vi "Wheel Pos Auto Adjust.vi"(7 "Action":enum16{"Initialize", "Analyzing", "Choosing"}(ring)=enum."Analyzing", 8 "error in":errorcluster, 10 "Wheel position":string, 11 "Refnum in":T2) -> (0 "error out":errorcluster, 1 "Best wheel position":string, 2 "No position match?":bool, 3 "Refnum out":T2, 4 "Laser position score":T1(array[cluster]))   [LabVIEW 2019, in "Image.lvlib"]
uses:
  Image.lvlib
  <vilib>/vision/Image Controls.llb/IMAQ Image.ctl
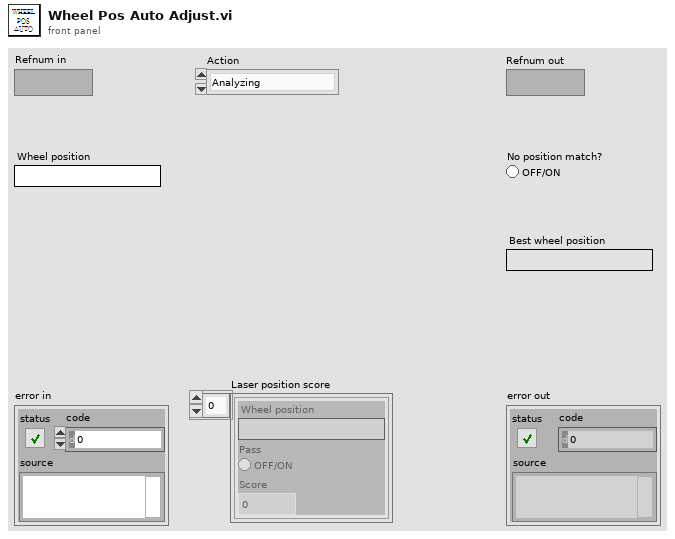
[diagram p1: front panel]
types:
  T1 = cluster{"Wheel position":string, "Pass":bool, "Score":i32}[]
  T2 = typedef "IMAQ Image.ctl" = refnum<image>
  T3 = cluster{"Laser position score":cluster{"Wheel position":string, "Pass":bool, "Score":i32}[], "No position match?":bool, "Best wheel position":string}
  T4 = cluster{"Wheel position":string, "Pass":bool, "Score":i32}
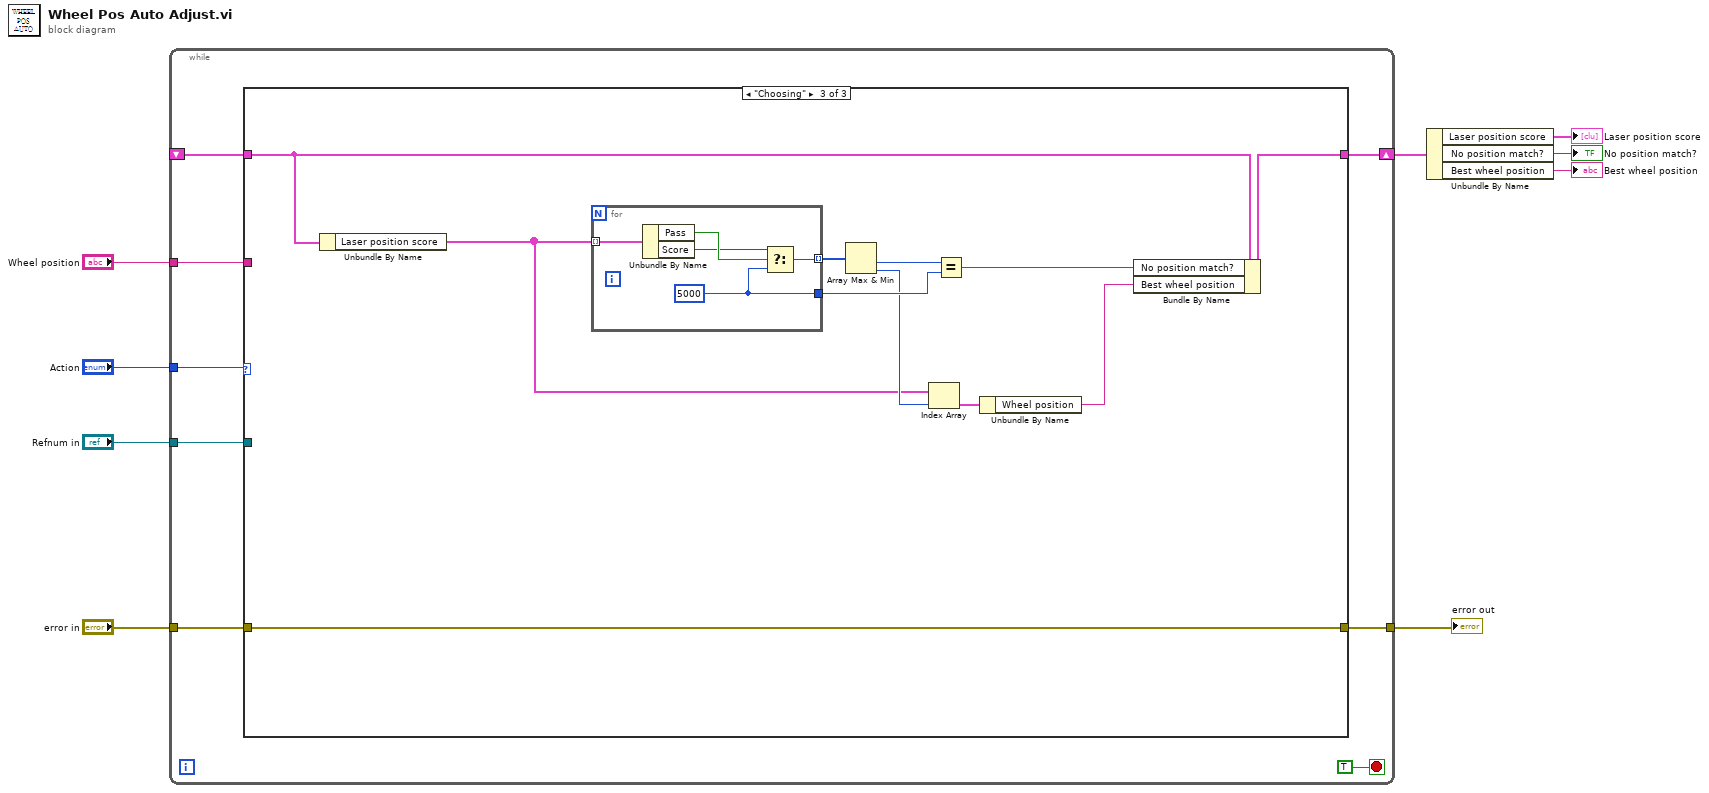
[diagram p0: block diagram]
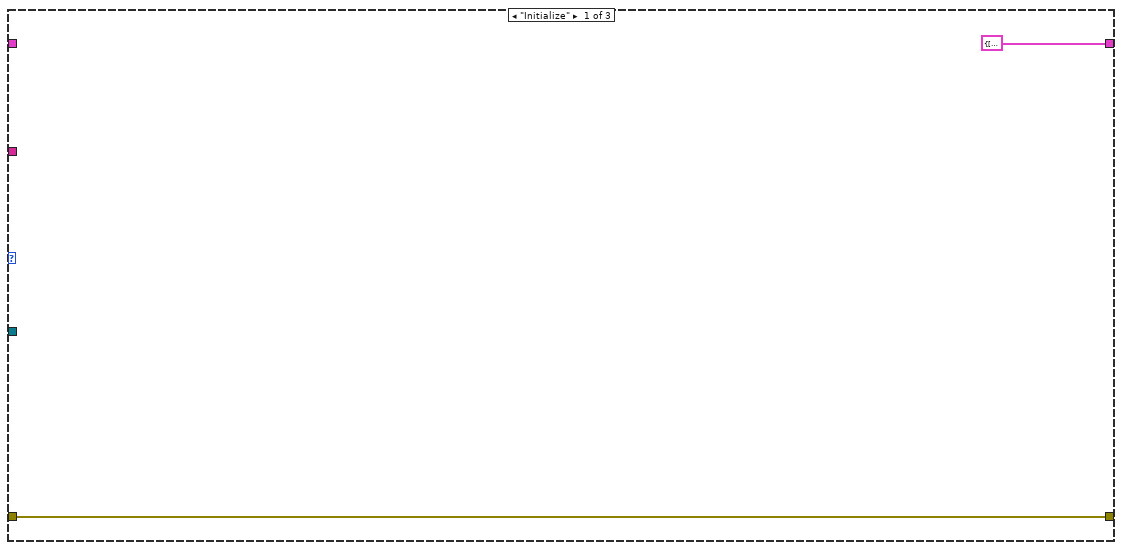
[diagram p2: hidden frame]
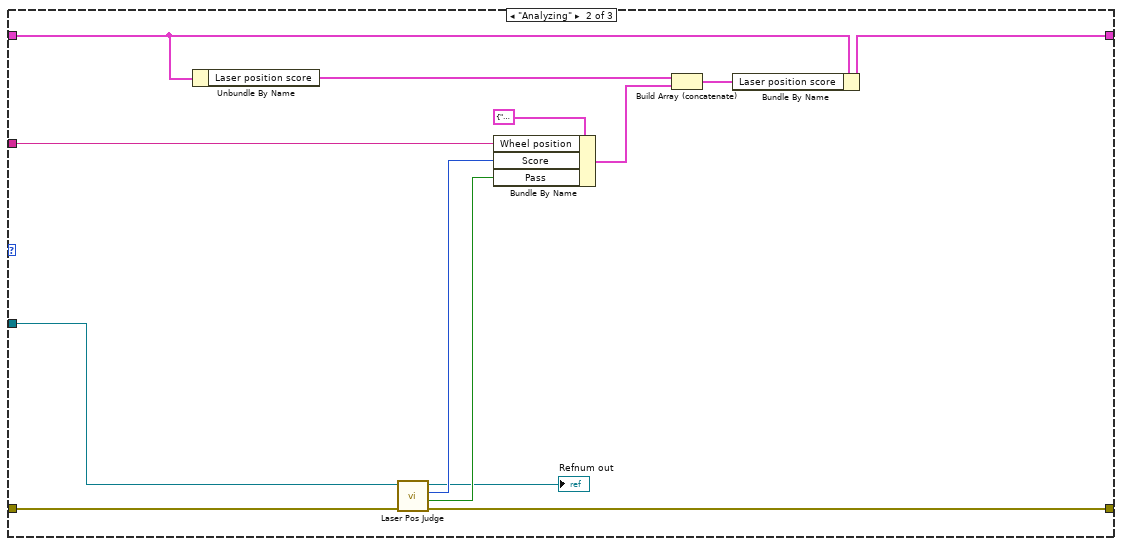
[diagram p3: hidden frame]
diagram:
  n1 = while {
    tunnel: "Action" -> [w17]
    tunnel: "Refnum in" -> [w16]
    shift-right: [w13] -> w4
    shift-left: _ -> [w14]
    tunnel: "error in" -> [w12]
    tunnel: "Wheel position" -> [w11]
    tunnel: [w10] -> w5
    stop <- TRUE stop-if-true
    n2 = case shown="\"Choosing\"" w17 {
      tunnel: w16 -> [_ w32 _]
      tunnel: w14 -> [_ w25 w37]
      tunnel: [T3 {"Laser position score"=[], "No position match?"=FALSE, "Best wheel position"=""} w22 w35] -> w13
      tunnel: w12 -> [w19 w29 w38]
      tunnel: w11 -> [_ w28 _]
      tunnel: [w19 w27 w38] -> w10
      frame "Initialize" {
      }
      frame "Analyzing" {
        n3 = Unbundle By Name(w25) -> ("Laser position score"=w24:T1)
        n4 = call "Laser Pos Judge.vi"("error in (no error)"=w29, "Refnum in"=w32) -> ("error out"=w27:errorcluster, "Boolean"=w31:bool, "Absolute R-L Score"=w30:i32, "Refnum out"=→"Refnum out":T2)  [unwired: 6 in]
        n5 = Bundle By Name(cluster=T4 {"Wheel position"="", "Pass"=TRUE, "Score"=0}, "Wheel position"=w28, "Score"=w30, "Pass"=w31) -> (w26:T4)
        n6 = Build Array (concatenate)(w24, w26) -> (w21:T1)
        n7 = Bundle By Name(cluster=w25, "Laser position score"=w21) -> (w22:T3)
      }
      frame "Choosing" {
        n8 = Unbundle By Name(w37) -> ("Laser position score"=w36:T1)
        n9 = for {
          tunnel: w36 -> [w48] mode=indexing
          tunnel: [w45] -> w43 mode=indexing
          tunnel: [w44] -> w41
          w44 = 5000 ("f")
          n10 = Unbundle By Name(w48) -> ("Pass"=w47:bool, "Score"=w46:i32)
          n11 = Select(t=w46, s=w47, f=w44) -> (s? t:f=w45:i32)
        }
        n12 = Array Max & Min(array=w43) -> (min value=w42:i32, min index (indices)=w40:i32)  [unwired: 2 out]
        n13 = Index Array(array=w36, index=w40) -> (element=w39:T4)
        n14 = Equal?(x=w42, y=w41) -> (x = y?=w34:bool)
        n15 = Unbundle By Name(w39) -> ("Wheel position"=w33:string)
        n16 = Bundle By Name(cluster=w37, "No position match?"=w34, "Best wheel position"=w33) -> (w35:T3)
      }
    }
  }
  "error out" <- w5
  n17 = Unbundle By Name(w4) -> ("Laser position score"=→"Laser position score":T1, "No position match?"=→"No position match?":bool, "Best wheel position"=→"Best wheel position":string)
